vi "Process.vi"(8 "error in":errorcluster, 11 "VoltageUpdateUI":refnum<class "VoltageUpdateUI.lvclass">) -> (0 "error out":errorcluster, 3 "VoltageUpdateUI out":refnum<class "VoltageUpdateUI.lvclass">)   [LabVIEW 2016, in "VoltageUpdateUI.lvclass"]
doc: "---------------------------------------------------------------\nJKI State Machine Objects™\nhttp://jki.net/state-machine-objects/\nCopyright (C) 2005-2015, JKI <info@jki.net>\nALL RIGHTS RESERVEDJKI State Machine Objects (SMO) 1.0.0.5\nJKI - JKI\nCopyright (c) 2016, JKI"
uses:
  VoltageUpdateUI.lvclass
  C:/Program Files (x86)/National Instruments/LabVIEW 2016/vi.lib/JKI/JKI SMO/SMO/SMO.lvclass
  C:/Program Files (x86)/National Instruments/LabVIEW 2016/vi.lib/JKI/JKI SMO/SMO.UI/SMO.UI.lvclass
  <vilib>/JKI/JKI SMO/SMO/Typedefs/Parent Call--Enum.ctl
  VoltageUpdateUI.lvclass/VoltageUpdateUI.ctl
  Program Files (x86)/National Instruments/LabVIEW 2016/templates/JKI/JKI SMO/Example Instrument/Typedefs/ExampleInstrument.getAll--Cluster.ctl
  <vilib>/JKI/JKI SMO/SMO.UI/SMO.UI.lvclass
  <userlib>/LevyLab/Levylab Instruments/SMOs/Instrument/Instrument.lvclass
  <vilib>/JKI/JKI SMO/SMO/SMO.lvclass
  Program Files (x86)/National Instruments/LabVIEW 2016/templates/JKI/JKI SMO/Example Instrument/ExampleInstrument.lvclass
panel:
  out "Numeric":u32
  out "Instrument Response":dbl
  in  "Set Parameter":bool
  in  "Parameter":dbl
  in  "STOP":bool
  out "SMO string":string
  out "SMO Boolean":bool
  out "Logger SMO":dbl
  out "Levy 1":dbl
  # "#todo\nmake UI here. maybe include a nice picture of the hardware?"
  # "#todo\nadd buttons to do stuff (e.g., change a setting)\nButtons should trigger an event"
  # "#todo\nresize this box if you want your UI to be different size"
  # "SMO UI Template"
  # "For instructions on how to use the JKI State Machine Objects, examples and video tutorials, visit:\nhttp://jki.net/state-machine-objects/\n\nJKI State Machine Objects™\nhttp://jki.net/state-machine-objects/\nCopyright (C) 2005-2015, JKI <info@jki.net>\nALL RIGHTS RESERVED"
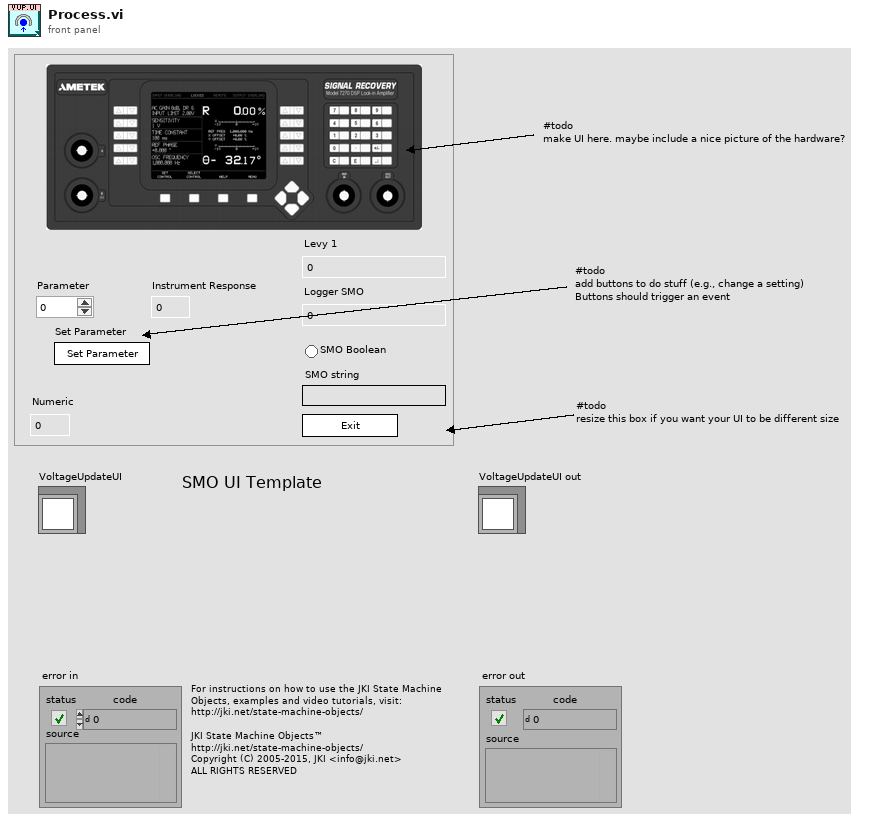
[diagram p1: front panel]
types:
  T1 = typedef "SMO.lvclass/Parent Call--Enum.ctl" = enum16{"Allows parent to run", "Does not request parent to run"}
  T2 = enum32{"invalid app kind", "Development System", "Run Time System", "Student Edition", "Embedded LabVIEW", "Evaluation", "Custom"}
  T3 = enum32{"Invalid", "Standard", "Closed", "Hidden", "Minimized", "Maximized"}
  T4 = typedef "ExampleInstrument.lvclass/ExampleInstrument.getAll--Cluster.ctl" = cluster{"Levy 1":dbl, "Logger SMO":dbl, "SMO Boolean":bool, "SMO String":string}
  T5 = cluster{"Core":cluster{"Current VI Reference":refnum<vi>, "Close Panel on Exit?":bool, "error":errorcluster}, "Self Reference":refnum<class "VoltageUpdateUI.lvclass">, "Instrument":refnum<class "Instrument.lvclass">, "getAll":variant, "Parameter":dbl}
  T6 = cluster{"Current VI Reference":refnum<vi>, "Close Panel on Exit?":bool, "error":errorcluster}
  T7 = typedef "SMO.lvclass/Protected Events.ctl" = cluster{"StopProcesses":refnum<user-event>, "AbortProcesses":refnum<user-event>, "Config Changed":refnum<user-event>, "Dependency":refnum<user-event>}
  T8 = typedef "Instrument.lvclass/PublicEvents--Cluster.ctl" = cluster{"MessageFromProcess":refnum<user-event>}
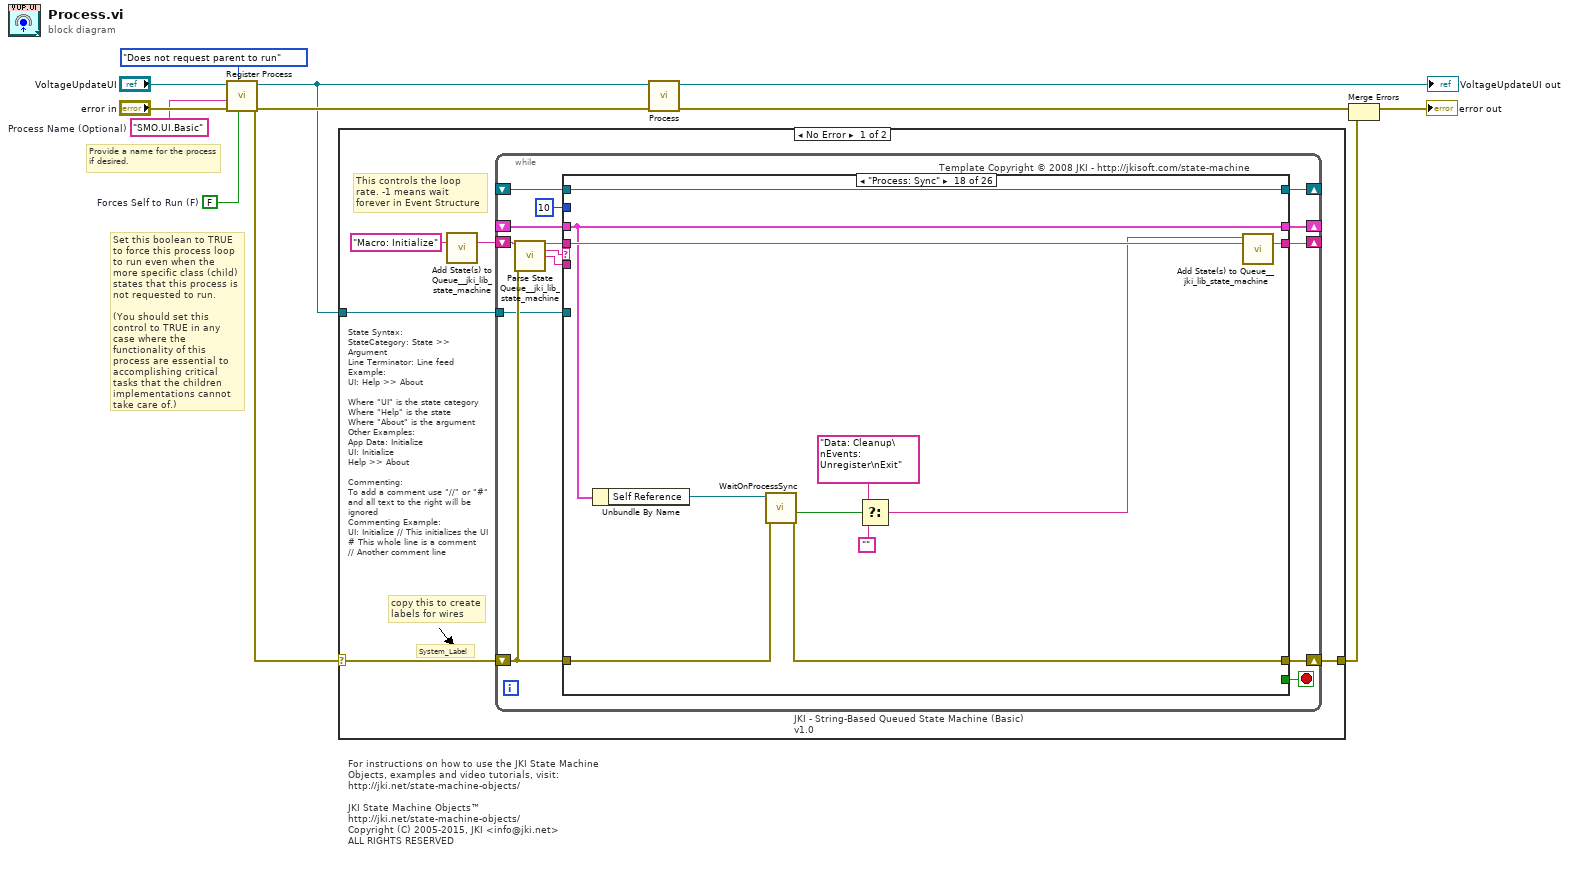
[diagram p0: block diagram]
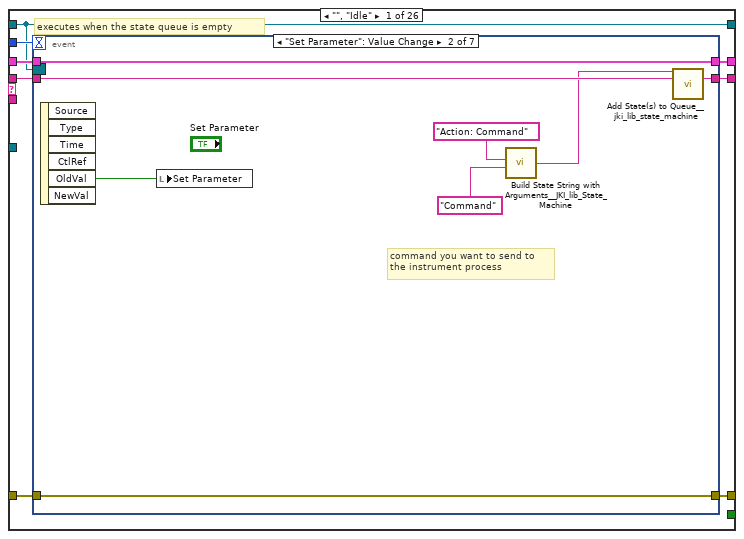
[diagram p2: hidden frame]
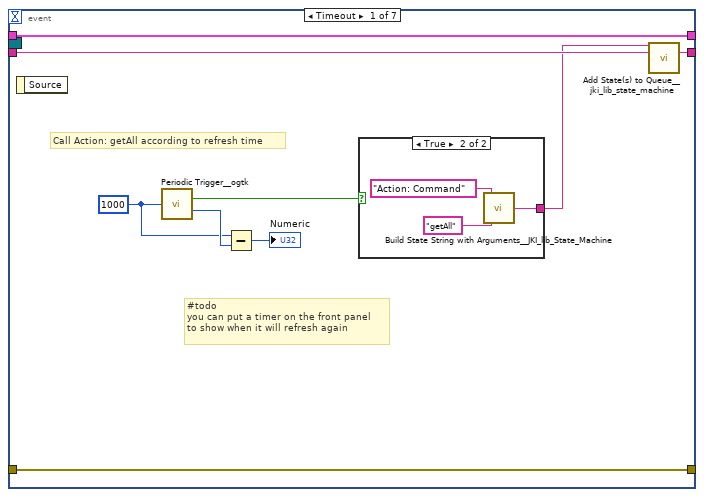
[diagram p3: hidden frame]
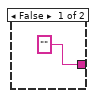
[diagram p4: hidden frame]
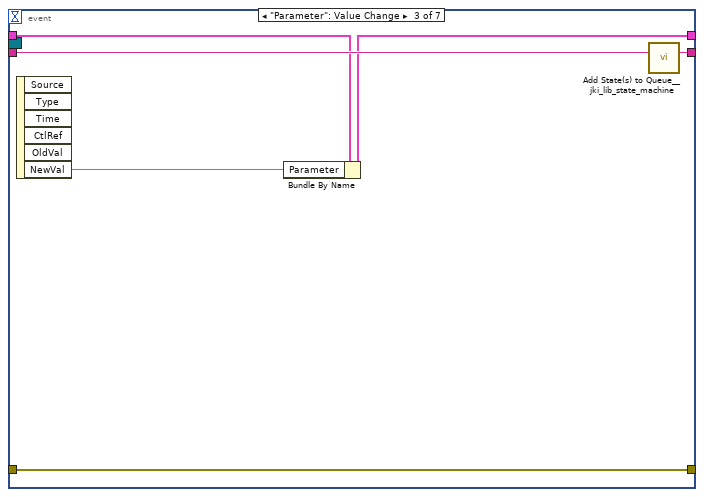
[diagram p5: hidden frame]
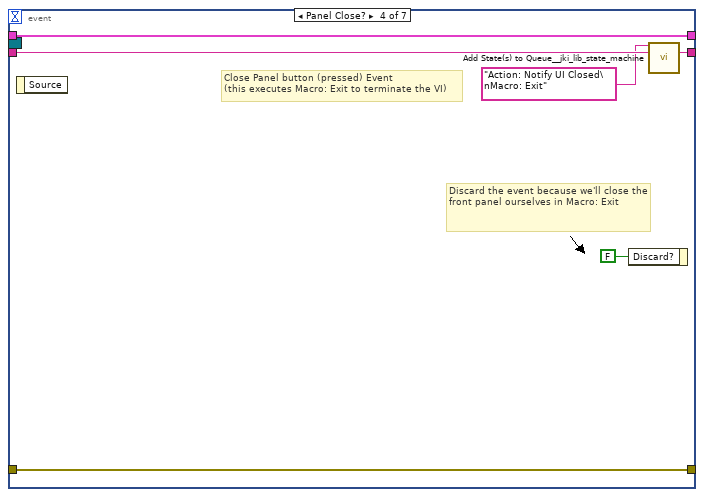
[diagram p6: hidden frame]
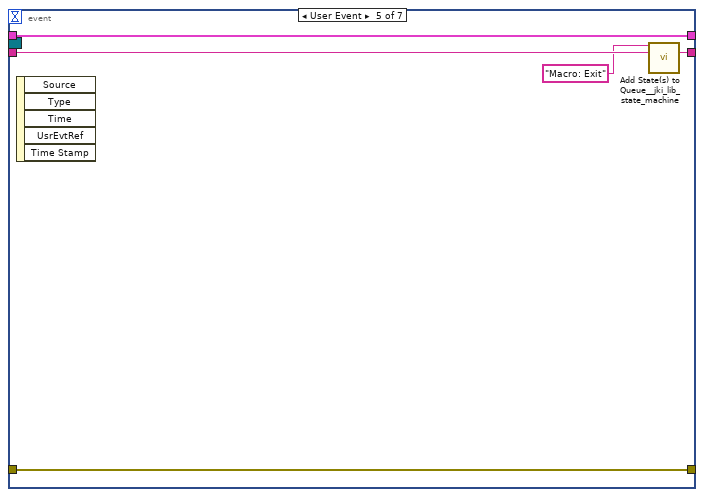
[diagram p7: hidden frame]
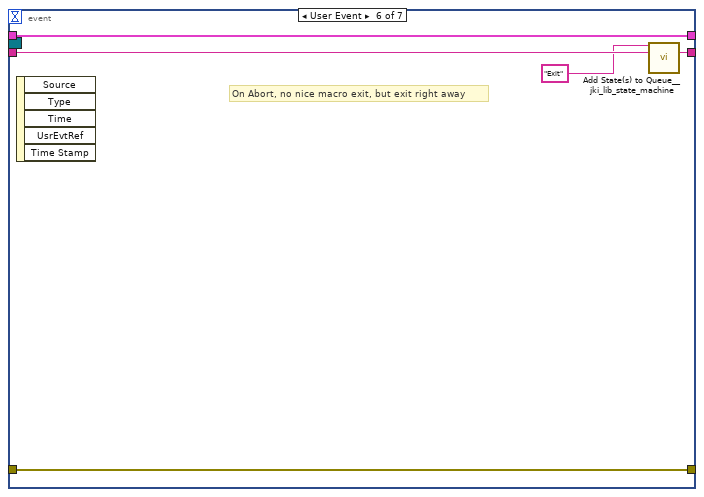
[diagram p8: hidden frame]
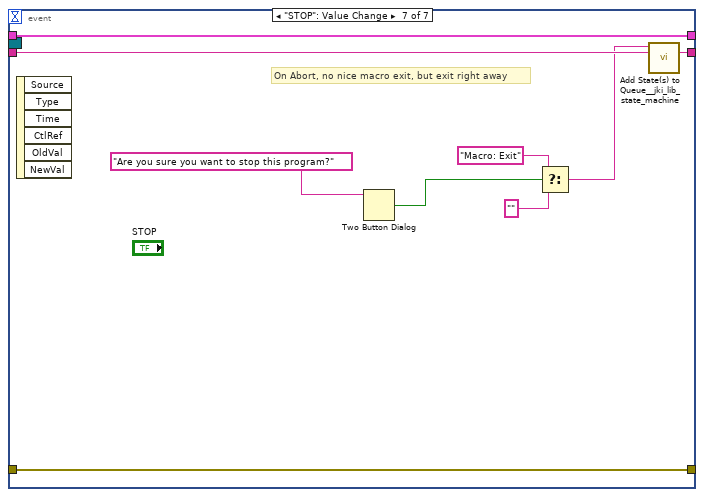
[diagram p9: hidden frame]
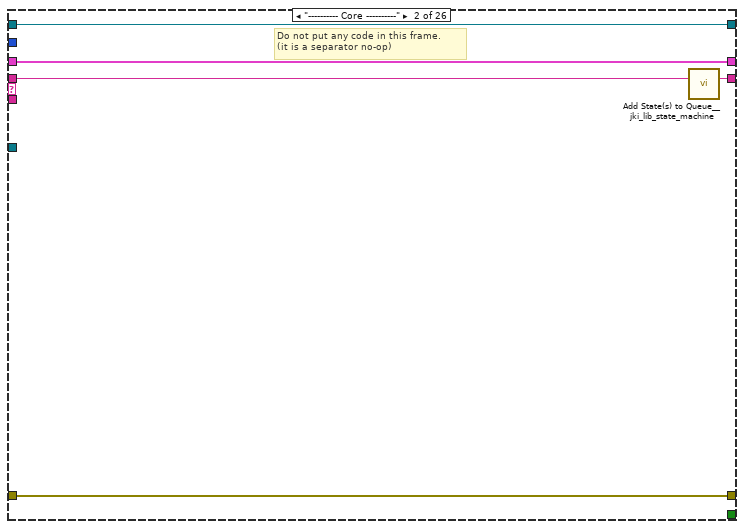
[diagram p10: hidden frame]
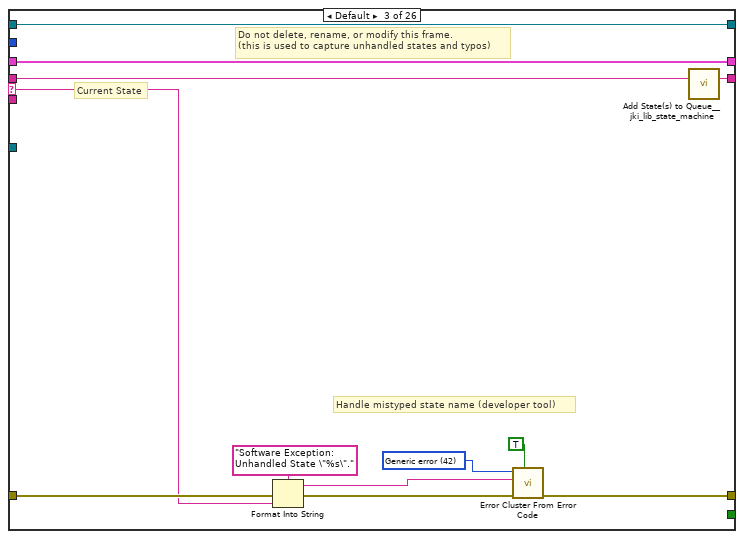
[diagram p11: hidden frame]
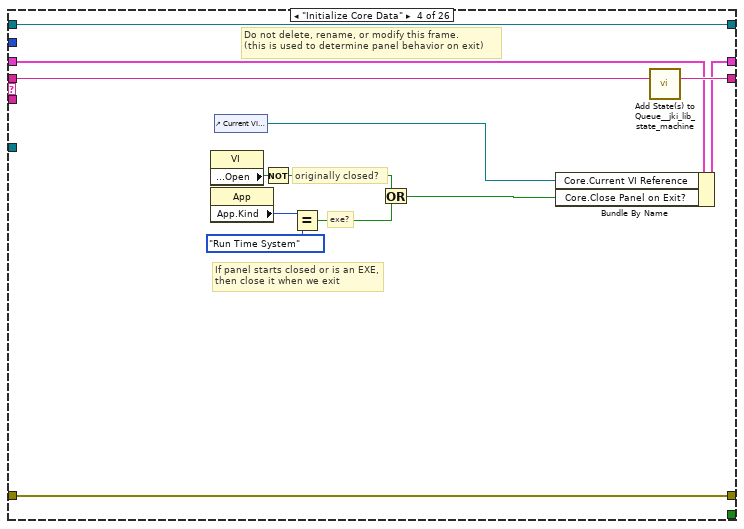
[diagram p12: hidden frame]
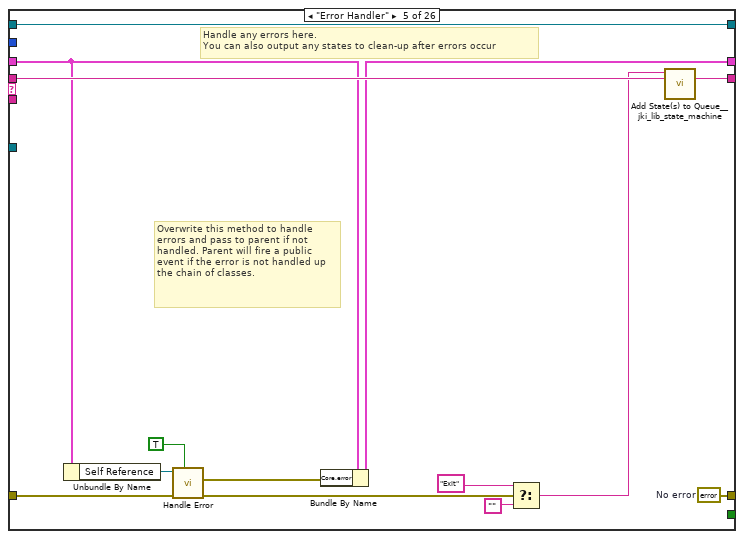
[diagram p13: hidden frame]
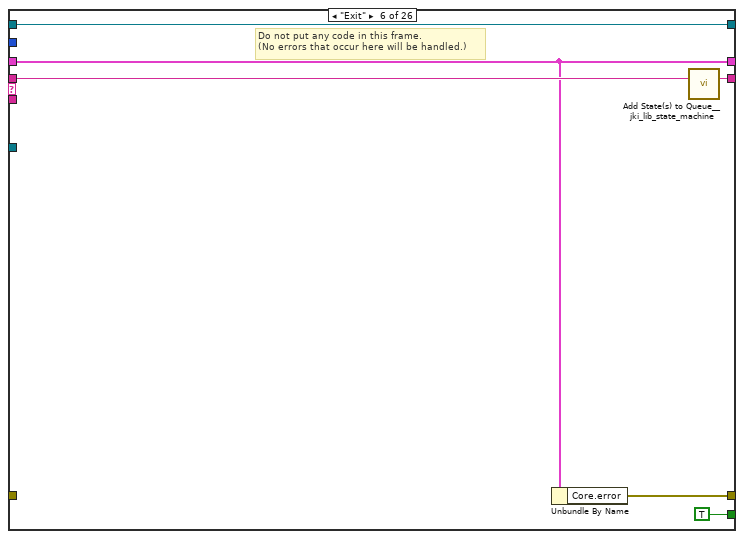
[diagram p14: hidden frame]
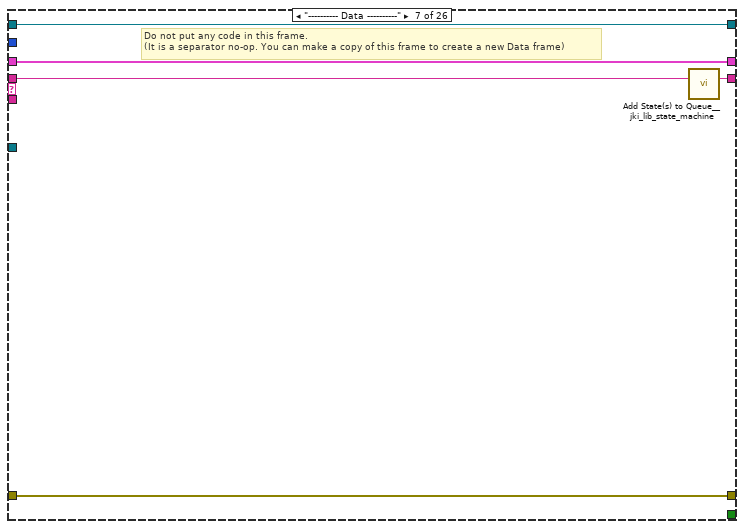
[diagram p15: hidden frame]
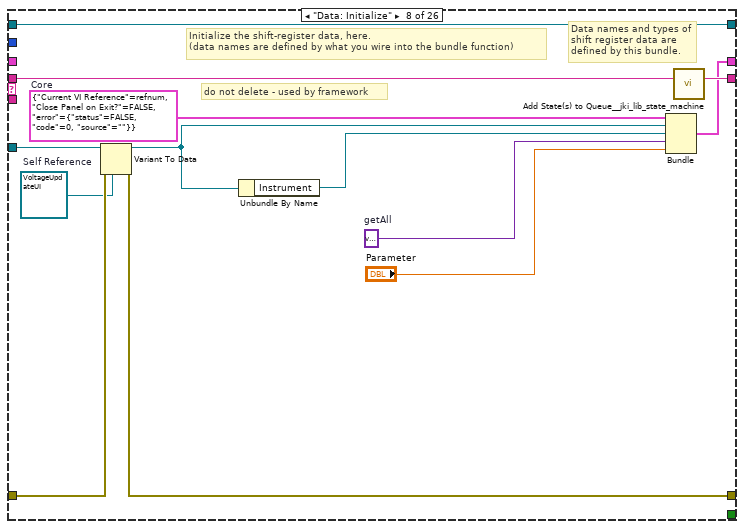
[diagram p16: hidden frame]
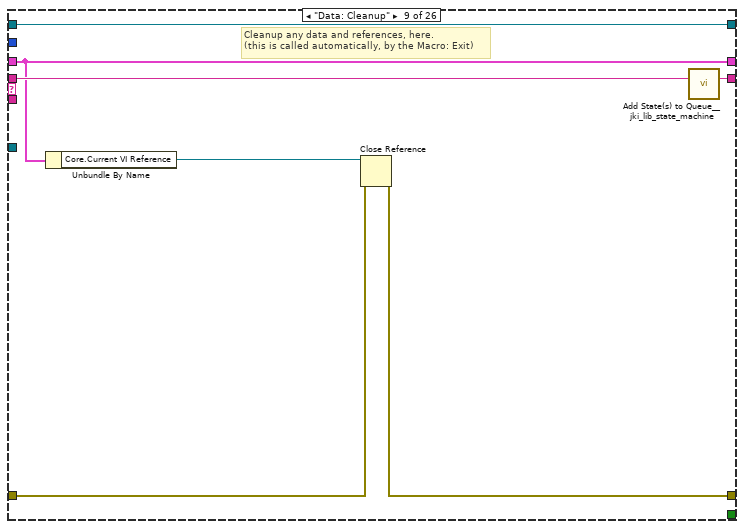
[diagram p17: hidden frame]
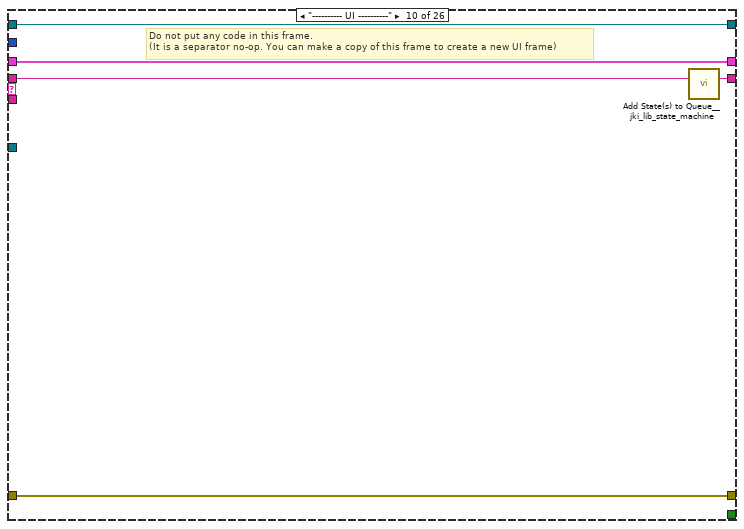
[diagram p18: hidden frame]
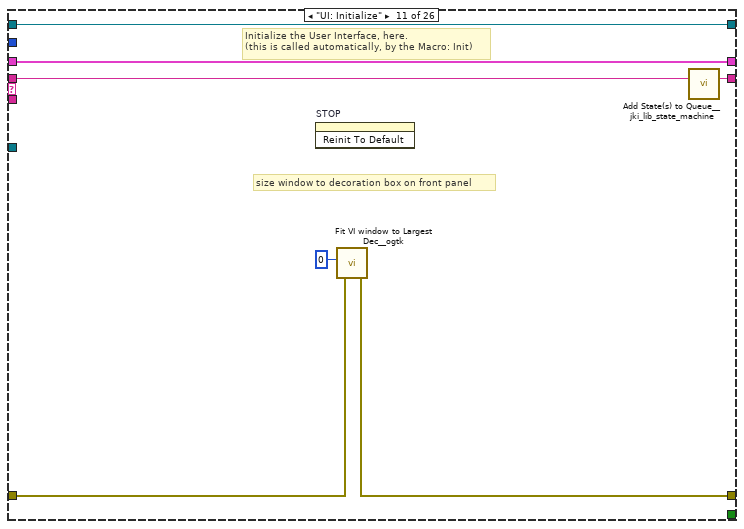
[diagram p19: hidden frame]
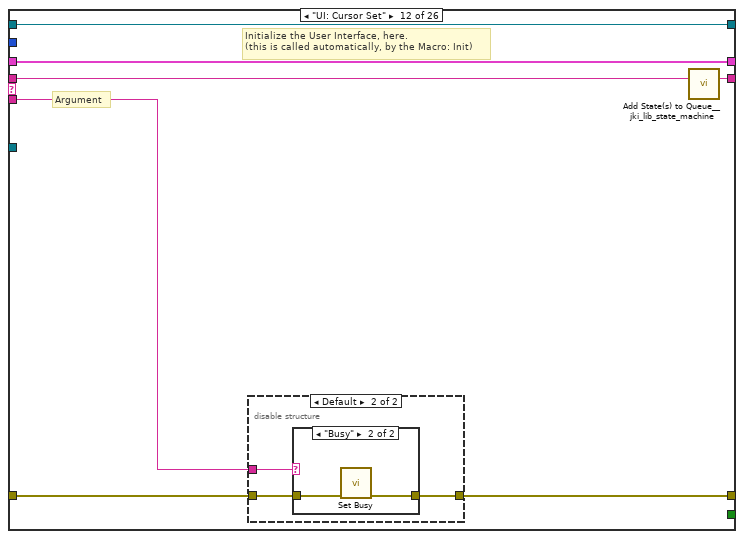
[diagram p20: hidden frame]
diagram:
  w2 = FALSE  # Forces Self to Run (F)
  w1 = "SMO.UI.Basic"  # Process Name (Optional)
  # "Provide a name for the process\nif desired."
  # "Set this boolean to TRUE to force this process loop to run even when the more specific class (child) states that this process is not requested to run.\n\n(You should set this control to TRUE in any case where the functionality of this process are essential to accomplishing critical tasks that the children implementations cannot take care of.)"
  # "For instructions on how to use the JKI State Machine Objects, examples and video tutorials, visit:\nhttp://jki.net/state-machine-objects/\n\nJKI State Machine Objects™\nhttp://jki.net/state-machine-objects/\nCopyright (C) 2005-2015, JKI <info@jki.net>\nALL RIGHTS RESERVED"
  n1 = call <vilib>:"Register Process.vi"("Forces Self to Run (F)"=w2, "Parent Call"=Parent_Call--Enum."Does not request parent to run", "error in (no error)"="error in", "Process Name (optional)"=w1, "SMO"="VoltageUpdateUI") -> ("error out"=w8:errorcluster, "SMO out"=w7:refnum<class "VoltageUpdateUI.lvclass">)  [unwired: 5 in]
  n2 = case shown="No Error" w8 {
    selector: w8 -> [w13 w368]
    tunnel: w7 -> [w14 _]
    tunnel: [w12 w368] -> w4
    frame No Error {
      # "State Syntax:\nStateCategory: State >> Argument\nLine Terminator: Line feed\nExample:\nUI: Help >> About\n\nWhere \"UI\" is the state category\nWhere \"Help\" is the state\nWhere \"About\" is the argument\nOther Examples:\nApp Data: Initialize\nUI: Initialize\nHelp >> About\n\nCommenting:\nTo add a comment use \"//\" or \"#\" and all text to the right will be ignored\nCommenting Example:\nUI: Initialize // This initializes the UI\n# This whole line is a comment\n// Another comment line"
      # "copy this to create labels for wires"
      # "This controls the loop rate. -1 means wait forever in Event Structure"
      # "System_Label"
      n3 = call <vilib>:"Add State(s) to Queue__jki_lib_state_machine.vi"("State(s) in (\"\")"="Macro: Initialize") -> ("States Out"=w16:string)  [unwired: 14 in]
      n4 = while "JKI - String-Based Queued State Machine (Basic) v1.0" {
        shift-right: [w23] -> _
        shift-left: _ -> [w22]
        shift-right: [w26] -> w12
        shift-left: w13 -> [w20]
        shift-right: [w25] -> _
        shift-left: w16 -> [w27]
        tunnel: w14 -> [w19]
        shift-right: [w18] -> _
        shift-left: _ -> [w17]
        stop <- w24 stop-if-true
        # "Template Copyright © 2008 JKI - http://jkisoft.com/state-machine"
        n5 = call <vilib>:"Parse State Queue__jki_lib_state_machine.vi"("State Queue"=w27, "Error In (no error)"=w20) -> ("Remaining States"=w29:string, "Current State"=w30:string, "Arguments"=w28:string)  [unwired: 11 in]
        n6 = case shown="\"Process: Sync\"" w30 {
          selector: w30 -> [_ _ w97 _ _ _ _ _ _ _ _ _ _ _ _ _ _ _ _ _ _ _ _ _ _ _]
          tunnel: w29 -> [w38 w95 w101 w120 w134 w140 w145 w158 w165 w170 w177 w184 w200 w232 w241 w255 w260 w271 w278 w283 w296 w302 w309 w316 w329 w348]
          tunnel: w28 -> [_ _ _ _ _ _ _ _ _ _ _ w178 w194 _ _ _ _ _ _ _ _ _ _ _ _ w336]
          tunnel: w22 -> [w36 w92 w99 w111 w123 w136 w142 _ w160 w167 w175 w182 w196 w229 w237 w246 w257 w268 w273 w280 w294 w300 w305 w312 w326 w345]
          tunnel: [w35 w93 w103 w117 w125 w135 w143 w154 w161 w168 w172 w179 w197 w230 w239 w253 w258 w262 w274 w281 w289 w297 w306 w310 w322 w338] -> w26
          tunnel: w20 -> [w34 w93 w102 w117 w130 _ w143 w155 w162 w168 w173 w180 w198 w230 w239 w253 w258 w263 w275 w281 w291 w298 w306 w311 w323 w339]
          tunnel: [w37 w94 w100 w119 w133 w139 w144 w157 w164 w169 w176 w183 w199 w231 w240 w254 w259 w270 w277 w282 w295 w301 w308 w315 w328 w347] -> w25
          tunnel: [_ _ _ _ _ TRUE _ _ _ _ _ _ _ _ _ _ _ _ _ _ _ _ _ _ _ _] -> w24
          tunnel: [w33 w92 w99 w118 w122 w136 w142 w156 w160 w167 w175 w182 w196 w229 w237 w246 w257 w268 w273 w280 w294 w300 w304 w312 w326 w342] -> w23
          tunnel: 10 ("Timeout") -> [w32 _ _ _ _ _ _ _ _ _ _ _ _ _ _ _ _ _ _ _ _ _ _ _ _ _]
          tunnel: w19 -> [_ _ _ _ _ _ _ w152 _ _ _ _ _ _ _ _ _ _ _ _ _ _ _ _ _ _]
          tunnel: [w31 w91 w96 w108 w132 w137 w141 w151 w159 w166 w174 w181 w193 w228 w238 w247 w256 w269 w276 w279 w293 w299 w307 w314 w327 w346] -> w18
          tunnel: w17 -> [w31 w91 w96 w108 w132 w137 w141 w151 w159 w166 w174 w181 w193 w228 w238 w247 w256 w269 w276 w279 _ w299 w307 w314 w327 w346]
          frame "", "Idle" {
            # "executes when the state queue is empty"
            n7 = event shown="[1] \"Set Parameter\": Value Change" {
              selector: w31 -> [_ _ _ _ _ _ _]
              dyn-events: _ -> [_ _ _ _ _ _ _]
              timeout: w32 -> [_ _ _ _ _ _ _]
              tunnel: w38 -> [w47 w59 w65 w71 w76 w81 w90]
              tunnel: [w46 w58 w64 w70 w75 w80 w89] -> w37
              tunnel: w36 -> [w44 w56 w61 w67 w73 w78 w87]
              tunnel: [w45 w57 w63 w66 w74 w79 w88] -> w35
              tunnel: w34 -> [w45 w57 w63 w66 w74 w79 w88]
              tunnel: [w44 w56 w60 w67 w73 w78 w87] -> w33
              event Timeout {
                w39 = u32 1000 ("time (ms)")
                # "#todo\nyou can put a timer on the front panel\nto show when it will refresh again"
                # "Call Action: getAll according to refresh time"
                n8 = event-data() -> ()  [unwired: 1 in, 1 out]
                n9 = call <userlib>:"Periodic Trigger__ogtk.vi"("time (ms)"=w39) -> ("Triggered"=w42:bool, "timer value"=w40:u32)  [unwired: 12 in, 1 out]
                n10 = Subtract(x=w39, y=w40) -> (x-y=→"Numeric":u32)
                n11 = case shown="True" w42 {
                  tunnel: ["" ("State(s) in Front (\"\")") w49] -> w43
                  frame False {
                  }
                  frame True {
                    n12 = call <vilib>:"Build State String with Arguments__JKI_lib_State_Machine.vi"("Arguments (\"\")"="getAll" ("State(s) in Front (\"\")"), "State"="Action: Command" ("State(s) in Front (\"\")")) -> ("State with Arguments"=w49:string)  [unwired: 4 in]
                  }
                }
                n13 = call <vilib>:"Add State(s) to Queue__jki_lib_state_machine.vi"("State(s) in Front (\"\")"=w43, "State(s) in (\"\")"=w47) -> ("States Out"=w46:string)  [unwired: 13 in]
              }
              event "Set Parameter": Value Change {
                # "command you want to send to\nthe instrument process"
                n14 = event-data() -> ("OldVal"=w55:bool)  [unwired: 1 in, 5 out]
                n15 = local write "Set Parameter"(w55) -> ()
                n16 = call <vilib>:"Build State String with Arguments__JKI_lib_State_Machine.vi"("Arguments (\"\")"="Command" ("State(s) in Front (\"\")"), "State"="Action: Command" ("State(s) in Front (\"\")")) -> ("State with Arguments"=w52:string)  [unwired: 4 in]
                n17 = call <vilib>:"Add State(s) to Queue__jki_lib_state_machine.vi"("State(s) in Front (\"\")"=w52, "State(s) in (\"\")"=w59) -> ("States Out"=w58:string)  [unwired: 13 in]
              }
              event "Parameter": Value Change {
                n18 = event-data() -> ("NewVal"=w62:dbl)  [unwired: 1 in, 5 out]
                n19 = Bundle By Name(cluster=w61, "Parameter"=w62) -> (w60:T5)
                n20 = call <vilib>:"Add State(s) to Queue__jki_lib_state_machine.vi"("State(s) in (\"\")"=w65) -> ("States Out"=w64:string)  [unwired: 14 in]
              }
              event Panel Close? {
                # "Discard the event because we'll close the front panel ourselves in Macro: Exit"
                # "Close Panel button (pressed) Event\n(this executes Macro: Exit to terminate the VI)"
                n21 = event-data() -> ()  [unwired: 1 in, 1 out]
                n22 = event-data("Discard?"=FALSE) -> ()  [unwired: 1 in, 1 out]
                n23 = call <vilib>:"Add State(s) to Queue__jki_lib_state_machine.vi"("State(s) in Front (\"\")"="Action: Notify UI Closed\nMacro: Exit", "State(s) in (\"\")"=w71) -> ("States Out"=w70:string)  [unwired: 13 in]
              }
              event User Event {
                n24 = event-data() -> ()  [unwired: 1 in, 5 out]
                n25 = call <vilib>:"Add State(s) to Queue__jki_lib_state_machine.vi"("State(s) in Front (\"\")"="Macro: Exit", "State(s) in (\"\")"=w76) -> ("States Out"=w75:string)  [unwired: 13 in]
              }
              event User Event {
                # "On Abort, no nice macro exit, but exit right away"
                n26 = event-data() -> ()  [unwired: 1 in, 5 out]
                n27 = call <vilib>:"Add State(s) to Queue__jki_lib_state_machine.vi"("State(s) in Front (\"\")"="Exit", "State(s) in (\"\")"=w81) -> ("States Out"=w80:string)  [unwired: 13 in]
              }
              event "STOP": Value Change {
                # "On Abort, no nice macro exit, but exit right away"
                n28 = event-data() -> ()  [unwired: 1 in, 6 out]
                n29 = Two Button Dialog(message="Are you sure you want to stop this program?") -> (T button?=w86:bool)  [unwired: 2 in]
                n30 = Select(t="Macro: Exit", s=w86, f="") -> (s? t:f=w82:string)
                n31 = call <vilib>:"Add State(s) to Queue__jki_lib_state_machine.vi"("State(s) in Front (\"\")"=w82, "State(s) in (\"\")"=w90) -> ("States Out"=w89:string)  [unwired: 13 in]
              }
            }
          }
          frame "---------- Core ----------" {
            # "Do not put any code in this frame.\n(it is a separator no-op)"
            n32 = call <vilib>:"Add State(s) to Queue__jki_lib_state_machine.vi"("State(s) in (\"\")"=w95) -> ("States Out"=w94:string)  [unwired: 14 in]
          }
          frame Default {
            w106 = 42 items=["No error", "Argument error", "Memory is full", "Out of zone", "End of file", "File already open", "Generic file I/O error", "File not found", "File permission error", "Disk is full", "Duplicate path", "Too many files open", "System feature not enabled", "Resource file not found", "Cannot add resource", "Resource not found", "Image not found", "Image memory error", "Pen does not exist", "Config type invalid", "Config token not found", "Config parse error", "Config memory error", "Bad external code format", "Bad external code offset", "External code not present", "Null window", "Destroy window error", "Null menu", "Print aborted", "Bad print record", "Print driver error", "Windows error during printing", "Memory error during printing", "Print dialog error", "Generic print error", "Invalid device refnum", "Device not found", "Device parameter error", "Device unit error", "Cannot open device", "Device call aborted", "Generic error", "Cancelled by user", "Object ID too low", "Object ID too high", "Object not in heap", "Unknown heap", "Unknown object (invalid DefProc)", "Unknown object (DefProc not in table)", "Message out of range", "Invalid (null) method", "Unknown message", "Manager call not supported", "Bad address", "Network operation in progress", "Network operation timed out", "Connection is busy", "Network attribute not supported", "Network error", "Address in use", "System out of memory", "Connection aborted", "Connection refused", "Not connected", "Already connected", "Connection closed", "Initialization error (interapplication manager)", "Bad occurrence", "Wait on unbound occurrence handler", "Occurrence queue overflow", "Datalog type conflict", "Unused", "Unrecognized type (interapplication manager)", "Memory corrupt", "Failed to make temporary DLL", "Old CIN version", "Drag socket not found", "Failed to load drop-object", "Failed to register OLE object", "Failed to release OLE object", "Format specifier type mismatch", "Unknown format specifier", "Too few format specifiers", "Too many format specifiers", "Scan failed", "Newer CIN version", "Error converting to variant", "Runtime menu error", "Password tampered", "Variant attribute not found", "Incompatible variant data type", "Event data is not available", "Event Store is not present", "Occurrence is not found", "Event Queue is not created", "Event info is not available", "Refnum passed is NULL", "Error retrieving Class GUID", "Error retrieving CoClass GUID", "Error retrieving TypeLib GUID.", "Bad built application magic bytes.", "Specific driver is different from the specific driver associated with the Logical Name.", "There is no session opened to the class driver.", "Max Error", "MAX - Error with config objects", "MAX - Error loading configuration", "MAX - Group not supported"]
            # "Current State"
            # "Do not delete, rename, or modify this frame.\n(this is used to capture unhandled states and typos)"
            # "Handle mistyped state name (developer tool)"
            n33 = Format Into String(format string="Software Exception: Unhandled State \"%s\"." ("message"), error in=w102, w97) -> (resulting string=w105:string, error out=w104:errorcluster)  [unwired: 1 in]
            n34 = call <vilib>:"Error Cluster From Error Code.vi"("show call chain? (False)"=TRUE, "error in (no error)"=w104, "error message (\"\")"=w105, "error code (0)"=w106) -> ("error out"=w103:errorcluster)  [unwired: 5 in]
            n35 = call <vilib>:"Add State(s) to Queue__jki_lib_state_machine.vi"("State(s) in (\"\")"=w101) -> ("States Out"=w100:string)  [unwired: 14 in]
          }
          frame "Initialize Core Data" {
            # "Do not delete, rename, or modify this frame.\n(this is used to determine panel behavior on exit)"
            # "originally closed?"
            # "exe?"
            # "If panel starts closed or is an EXE, then close it when we exit"
            n36 = property class="VI"() -> ("Front Panel.Open"=w116:bool)  [unwired: 2 in, 2 out]
            n37 = property class="App"() -> ("App.Kind"=w115:T2)  [unwired: 2 in, 2 out]
            n38 = control-ref of="Current VI Reference"() -> (w109:refnum<vi>)
            n39 = Not(x=w116) -> (.not. x?=w113:bool)
            n40 = Equal?(x=w115, y=T2."Run Time System" ("Application:Kind")) -> (x = y?=w112:bool)
            n41 = Or(x=w113, y=w112) -> (x .or. y?=w110:bool)
            n42 = Bundle By Name(cluster=w111, "Core.Current VI Reference"=w109, "Core.Close Panel on Exit?"=w110) -> (w118:T5)
            n43 = call <vilib>:"Add State(s) to Queue__jki_lib_state_machine.vi"("State(s) in (\"\")"=w120) -> ("States Out"=w119:string)  [unwired: 14 in]
          }
          frame "Error Handler" {
            w125 = errorcluster {"status"=FALSE, "code"=0, "source"=""}  # No error
            # "Overwrite this method to handle errors and pass to parent if not handled. Parent will fire a public event if the error is not handled up the chain of classes."
            # "Handle any errors here.\nYou can also output any states to clean-up after errors occur"
            n44 = Unbundle By Name(w123) -> ("Self Reference"=w131:refnum<class "VoltageUpdateUI.lvclass">)
            n45 = call-dynamic "Handle Error.vi"("Stop on Unhandled Error (T)"=TRUE, "error in"=w130, "SMO"=w131) -> ("handling error"=w126:errorcluster, "Unhandled error"=w124:errorcluster)  [unwired: 6 in, 1 out]
            n46 = Bundle By Name(cluster=w123, "Core.error"=w124) -> (w122:T5)
            n47 = Select(t="Exit", s=w126, f="") -> (s? t:f=w127:string)
            n48 = call <vilib>:"Add State(s) to Queue__jki_lib_state_machine.vi"("State(s) in Front (\"\")"=w127, "State(s) in (\"\")"=w134) -> ("States Out"=w133:string)  [unwired: 13 in]
          }
          frame "Exit" {
            # "Do not put any code in this frame.\n(No errors that occur here will be handled.)"
            n49 = Unbundle By Name(w136) -> ("Core.error"=w135:errorcluster)
            n50 = call <vilib>:"Add State(s) to Queue__jki_lib_state_machine.vi"("State(s) in (\"\")"=w140) -> ("States Out"=w139:string)  [unwired: 14 in]
          }
          frame "---------- Data ----------" {
            # "Do not put any code in this frame.\n(It is a separator no-op. You can make a copy of this frame to create a new Data frame)"
            n51 = call <vilib>:"Add State(s) to Queue__jki_lib_state_machine.vi"("State(s) in (\"\")"=w145) -> ("States Out"=w144:string)  [unwired: 14 in]
          }
          frame "Data: Initialize" {
            w147 = variant  # getAll
            w150 = T6 {"Current VI Reference"=refnum, "Close Panel on Exit?"=FALSE, "error"={"status"=FALSE, "code"=0, "source"=""}}  # Core
            w153 = refnum<class "VoltageUpdateUI.lvclass"> refnum  # Self Reference
            # "do not delete - used by framework"
            # "Data names and types of shift register data are defined by this bundle."
            # "Initialize the shift-register data, here.\n(data names are defined by what you wire into the bundle function)"
            n52 = Variant To Data(error in=w155, type=w153, Variant=w152) -> (data=w149:refnum<class "VoltageUpdateUI.lvclass">, error out=w154:errorcluster)
            n53 = Unbundle By Name(w149) -> ("Instrument"=w148:refnum<class "Instrument.lvclass">)
            n54 = Bundle("Core"=w150, "Self Reference"=w149, "Instrument"=w148, "getAll"=w147, "Parameter"="Parameter") -> (w156:T5)  [unwired: 1 in]
            n55 = call <vilib>:"Add State(s) to Queue__jki_lib_state_machine.vi"("State(s) in (\"\")"=w158) -> ("States Out"=w157:string)  [unwired: 14 in]
          }
          frame "Data: Cleanup" {
            # "Cleanup any data and references, here.\n(this is called automatically, by the Macro: Exit)"
            n56 = Unbundle By Name(w160) -> ("Core.Current VI Reference"=w163:refnum<vi>)
            n57 = Close Reference(reference=w163, error in (no error)=w162) -> (error out=w161:errorcluster)
            n58 = call <vilib>:"Add State(s) to Queue__jki_lib_state_machine.vi"("State(s) in (\"\")"=w165) -> ("States Out"=w164:string)  [unwired: 14 in]
          }
          frame "---------- UI ----------" {
            # "Do not put any code in this frame.\n(It is a separator no-op. You can make a copy of this frame to create a new UI frame)"
            n59 = call <vilib>:"Add State(s) to Queue__jki_lib_state_machine.vi"("State(s) in (\"\")"=w170) -> ("States Out"=w169:string)  [unwired: 14 in]
          }
          frame "UI: Initialize" {
            # "size window to decoration box on front panel"
            # "Initialize the User Interface, here.\n(this is called automatically, by the Macro: Init)"
            n60 = invoke on="STOP" class="Bool (strict)" method="Reinit To Default"() -> ()  [unwired: 3 in, 3 out]
            n61 = call <userlib>:"Fit VI window to Largest Dec__ogtk.vi"("error in (no error)"=w173, "border spacing (2 px)"=0) -> ("error out"=w172:errorcluster)  [unwired: 4 in, 1 out]
            n62 = call <vilib>:"Add State(s) to Queue__jki_lib_state_machine.vi"("State(s) in (\"\")"=w177) -> ("States Out"=w176:string)  [unwired: 14 in]
          }
          frame "UI: Cursor Set" {
            # "Argument"
            # "Initialize the User Interface, here.\n(this is called automatically, by the Macro: Init)"
            n63 = disable-structure shown="Default" {
              disable-tunnel: w180 -> [w185 w188]
              disable-tunnel: [w185 w187] -> w179
              disable-tunnel: w178 -> [_ w186]
              frame condition #0 {
              }
              frame condition #1 (active) {
                n64 = case shown="\"Busy\"" w186 {
                  tunnel: w188 -> [w190 w192]
                  tunnel: [w189 w191] -> w187
                  frame "Idle", Default {
                    n65 = call <vilib>:"Unset Busy.vi"("error in (no error)"=w190) -> ("error out"=w189:errorcluster)  [unwired: 10 in]
                  }
                  frame "Busy" {
                    n66 = call <vilib>:"Set Busy.vi"("error in (no error)"=w192) -> ("error out"=w191:errorcluster)  [unwired: 9 in, 1 out]
                  }
                }
              }
            }
            n67 = call <vilib>:"Add State(s) to Queue__jki_lib_state_machine.vi"("State(s) in (\"\")"=w184) -> ("States Out"=w183:string)  [unwired: 14 in]
          }
          frame "UI: Front Panel State" {
            # "Argument"
            # "Set Front Panel Open or Closed\n(Usage: \"UI: Front Panel State >> Open|Close\")"
            n68 = Unbundle By Name(w196) -> ("Core.Current VI Reference"=w195:refnum<vi>)
            n69 = disable-structure shown="Default" {
              disable-tunnel: w198 -> [w204 w227]
              disable-tunnel: [w203 w227] -> w197
              disable-tunnel: w195 -> [w202 _]
              disable-tunnel: w194 -> [w201 _]
              frame condition #0 (active) {
                n70 = case shown="\"Close\"" w201 {
                  tunnel: w204 -> [w208 w221]
                  tunnel: [w210 w222] -> w203
                  tunnel: w202 -> [w209 w219]
                  frame "Open", Default {
                    n71 = property class="VI"(reference=w209, error in=w208) -> (reference out=w206:refnum<vi>, error out=w207:errorcluster, "FP.State"=w205:T3)
                    n72 = case shown="\"Closed\"" w205 {
                      tunnel: [w213 w216] -> w210
                      tunnel: w207 -> [w212 w216]
                      tunnel: w206 -> [w211 _]
                      frame "Closed" {
                        n73 = invoke class="VI" method="FP.Open"(reference=w211, error in=w212, "Activate"=TRUE, "State"=T3."Standard") -> (error out=w213:errorcluster)  [unwired: 1 in, 4 out]
                      }
                      frame Default {
                      }
                    }
                  }
                  frame "Close" {
                    n74 = property class="VI"(reference=w219, error in=w221) -> (reference out=w218:refnum<vi>, error out=w220:errorcluster, "FP.State"=w217:T3)
                    n75 = case shown="Default" w217 {
                      tunnel: [w223 w226] -> w222
                      tunnel: w220 -> [w223 w225]
                      tunnel: w218 -> [_ w224]
                      frame "Invalid", "Closed" {
                      }
                      frame Default {
                        n76 = invoke class="VI" method="FP.Close"(reference=w224, error in=w225) -> (error out=w226:errorcluster)  [unwired: 1 in, 2 out]
                      }
                    }
                  }
                }
              }
              frame condition #1 {
              }
            }
            n77 = call <vilib>:"Add State(s) to Queue__jki_lib_state_machine.vi"("State(s) in (\"\")"=w200) -> ("States Out"=w199:string)  [unwired: 14 in]
          }
          frame "---------- Macro ----------" {
            # "Do not put any code in this frame.\n(It is a separator no-op. You can make a copy of this frame to create a new Macro frame)"
            n78 = call <vilib>:"Add State(s) to Queue__jki_lib_state_machine.vi"("State(s) in (\"\")"=w232) -> ("States Out"=w231:string)  [unwired: 14 in]
          }
          frame "Macro: Initialize" {
            w235 = "UI: Initialize\n//UI: Front Panel State >> Open"  # UI: Initialize //UI: Front Panel State >> Open
            # "Initialization Macro\n(This is called once, when the VI starts)"
            n79 = call <vilib>:"Add State(s) to Queue__jki_lib_state_machine.vi"("State(s) in Front (\"\")"="Data: Initialize\nInitialize Core Data\nEvents: Register", "State(s) in (\"\")"="Process: Sync", "State(s) at Back (\"\")"=w235) -> ("States Out"=w234:string)  [unwired: 12 in]
            n80 = call <vilib>:"Add State(s) to Queue__jki_lib_state_machine.vi"("State(s) in Front (\"\")"=w234, "State(s) in (\"\")"=w241) -> ("States Out"=w240:string)  [unwired: 13 in]
          }
          frame "Macro: Exit" {
            # "Exit Macro\n(This is called once, when the VI exits)"
            n81 = Unbundle By Name(w246) -> ("Core.Close Panel on Exit?"=w252:bool)
            n82 = Select(t="//UI: Front Panel State >> Close", s=w252, f="") -> (s? t:f=w249:string)
            n83 = call <vilib>:"Add State(s) to Queue__jki_lib_state_machine.vi"("State(s) in Front (\"\")"="Data: Cleanup\nEvents: Unregister\nProcess: Self Terminate", "State(s) in (\"\")"="Process: Sync", "State(s) at Back (\"\")"="Exit") -> ("States Out"=w243:string)  [unwired: 12 in]
            n84 = call <vilib>:"Add State(s) to Queue__jki_lib_state_machine.vi"("State(s) in (\"\")"=w249, "State(s) at Back (\"\")"=w243) -> ("States Out"=w248:string)  [unwired: 13 in]
            n85 = call <vilib>:"Add State(s) to Queue__jki_lib_state_machine.vi"("State(s) in Front (\"\")"=w248, "State(s) in (\"\")"=w255) -> ("States Out"=w254:string)  [unwired: 13 in]
          }
          frame "---------- Process ----------" {
            # "Template Separator\n(You can make a copy of, or modify, this frame)"
            n86 = call <vilib>:"Add State(s) to Queue__jki_lib_state_machine.vi"("State(s) in (\"\")"=w260) -> ("States Out"=w259:string)  [unwired: 14 in]
          }
          frame "Process: Sync" {
            n87 = Unbundle By Name(w268) -> ("Self Reference"=w264:refnum<class "VoltageUpdateUI.lvclass">)
            n88 = call <vilib>:"WaitOnProcessSync.vi"("error in (no error)"=w263, "SMO"=w264) -> ("error out"=w262:errorcluster, "Don't run?"=w267:bool)  [unwired: 7 in, 1 out]
            n89 = Select(t="Data: Cleanup\nEvents: Unregister\nExit", s=w267, f="") -> (s? t:f=w261:string)
            n90 = call <vilib>:"Add State(s) to Queue__jki_lib_state_machine.vi"("State(s) in Front (\"\")"=w261, "State(s) in (\"\")"=w271) -> ("States Out"=w270:string)  [unwired: 13 in]
          }
          frame "Process: Self Terminate" {
            n91 = Unbundle By Name(w273) -> ("Self Reference"=w272:refnum<class "VoltageUpdateUI.lvclass">)
            n92 = call <vilib>:"SelfTerminate.vi"("error in (no error)"=w275, "SMO in"=w272) -> ("error out"=w274:errorcluster)  [unwired: 8 in, 1 out]
            n93 = call <vilib>:"Add State(s) to Queue__jki_lib_state_machine.vi"("State(s) in (\"\")"=w278) -> ("States Out"=w277:string)  [unwired: 14 in]
          }
          frame "---------- Events ----------" {
            # "Template Separator\n(You can make a copy of, or modify, this frame)"
            n94 = call <vilib>:"Add State(s) to Queue__jki_lib_state_machine.vi"("State(s) in (\"\")"=w283) -> ("States Out"=w282:string)  [unwired: 14 in]
          }
          frame "Events: Register" {
            # "Expand to add\nmore events"
            # "Base Class Protected Events"
            n95 = Unbundle By Name(w294) -> ("Self Reference"=w287:refnum<class "VoltageUpdateUI.lvclass">, "Instrument"=w286:refnum<class "Instrument.lvclass">)
            n96 = call <vilib>:"GetProtectedEvents.vi"("SMO"=w287) -> ("error out"=w288:errorcluster, "SMO Protected Events"=w292:T7)  [unwired: 8 in, 1 out]
            n97 = call <userlib>:"Instrument.GetPublicEvents.vi"("Instrument"=w286) -> ("error out"=w284:errorcluster, "Instrument Public Events"=w285:T8)  [unwired: 8 in, 1 out]
            n98 = register-events(w292, w285) -> (reference out=w293:refnum<event-registration>, error out=w290:errorcluster)  [unwired: 2 in]
            n99 = Merge Errors(w284, w291, w290, w288) -> (w289:errorcluster)
            n100 = call <vilib>:"Add State(s) to Queue__jki_lib_state_machine.vi"("State(s) in (\"\")"=w296) -> ("States Out"=w295:string)  [unwired: 14 in]
          }
          frame "Events: Unregister" {
            n101 = Unregister For Events(event registration refnum=w299, error in=w298) -> (error out=w297:errorcluster)
            n102 = call <vilib>:"Add State(s) to Queue__jki_lib_state_machine.vi"("State(s) in (\"\")"=w302) -> ("States Out"=w301:string)  [unwired: 14 in]
          }
          frame "---------- Action ----------" {
            n103 = Unbundle By Name(w305) -> ("Self Reference"=w303:refnum<class "VoltageUpdateUI.lvclass">)
            n104 = Bundle By Name(cluster=w305, "Self Reference"=w303) -> (w304:T5)
            n105 = call <vilib>:"Add State(s) to Queue__jki_lib_state_machine.vi"("State(s) in (\"\")"=w309) -> ("States Out"=w308:string)  [unwired: 14 in]
          }
          frame "Action: Notify UI Closed" {
            # "Notify that the UI has been closed"
            n106 = Unbundle By Name(w312) -> ("Self Reference"=w313:refnum<class "VoltageUpdateUI.lvclass">)
            n107 = call <vilib>:"Hide.vi"("error in (no error)"=w311, "SMO.UI"=w313) -> ("error out"=w310:errorcluster)  [unwired: 8 in, 1 out]
            n108 = call <vilib>:"Add State(s) to Queue__jki_lib_state_machine.vi"("State(s) in (\"\")"=w316) -> ("States Out"=w315:string)  [unwired: 14 in]
          }
          frame "Action: Update Front Panel" {
            # "do this way to have nicer UI or only display what you want"
            # "typedef from Child Instrument"
            n109 = Unbundle By Name(w326) -> ("getAll"=w325:variant)
            n110 = Variant To Data(error in=w323, type=T4 {"Levy 1"=0.0, "Logger SMO"=0.0, "SMO Boolean"=FALSE, "SMO String"=""} ("getAll"), Variant=w325) -> (data=w321:T4, error out=w322:errorcluster)
            n111 = Unbundle By Name(w321) -> ("Levy 1"=→"Levy 1":dbl, "Logger SMO"=→"Logger SMO":dbl, "SMO Boolean"=→"SMO Boolean":bool, "SMO String"=→"SMO string":string)
            n112 = call <vilib>:"Add State(s) to Queue__jki_lib_state_machine.vi"("State(s) in (\"\")"=w329) -> ("States Out"=w328:string)  [unwired: 14 in]
          }
          frame "Action: Command" {
            # "#todo:\nconfigure here how to parse messages from Instrument"
            # "command"
            n113 = Unbundle By Name(w345) -> ("Self Reference"=w334:refnum<class "VoltageUpdateUI.lvclass">, "Instrument"=w332:refnum<class "Instrument.lvclass">, "Parameter"=w341:dbl)
            n114 = call-dynamic "Remote Client.vi"("Wait for Response?"=TRUE, "error in (no error)"=w339, "Data"=w341, "Command"=w336, "Instrument in"=w332) -> ("error out"=w340:errorcluster, "Data out"=w343:variant, "Command out"=w344:string)  [unwired: 3 in, 1 out]
            n115 = case shown="Default" w344 {
              tunnel: w343 -> [_ w355 w367]
              tunnel: w340 -> [w353 w358 w365]
              tunnel: [w353 w358 w363] -> w338
              tunnel: [w351 w357 w362] -> w335
              tunnel: w334 -> [w351 w357 w362]
              tunnel: ["" ("State(s) in Front (\"\")") "Action: Update Front Panel" ("State(s) in Front (\"\")") "" ("State(s) in Front (\"\")")] -> w333
              tunnel: w332 -> [w352 w354 w360]
              tunnel: [w352 w354 w360] -> w331
              tunnel: [variant ("Data out") w355 variant ("Data out")] -> w330
              frame Default {
              }
              frame "getAll" {
              }
              frame "setMagnet" {
                n116 = Variant To Data(error in=w365, type=0.0 ("Magnet Return"), Variant=w367) -> (data=→"Instrument Response":dbl, error out=w363:errorcluster)
              }
            }
            n117 = Bundle By Name(cluster=w345, "Self Reference"=w335, "Instrument"=w331, "getAll"=w330) -> (w342:T5)
            n118 = call <vilib>:"Add State(s) to Queue__jki_lib_state_machine.vi"("State(s) in Front (\"\")"=w333, "State(s) in (\"\")"=w348) -> ("States Out"=w347:string)  [unwired: 13 in]
          }
        }
      }
    }
    frame Error {
    }
  }
  n119 = call-parent "Process.vi"("error in (no error)"=w8, "SMO.UI"=w7) -> ("error out"=w5:errorcluster, "SMO.UI out"=→"VoltageUpdateUI out":refnum<class "VoltageUpdateUI.lvclass">)  [unwired: 8 in]
  n120 = Merge Errors(w5, w4) -> (→"error out":errorcluster)
